vi "state_to_pose.vi"(1 "Handle State":sgl[][](array[numeric])) -> (0 "Pose":T1)   [LabVIEW 2013]
uses:
  <vilib>/Analysis/Matrix/Datatypes/RealMatrix.ctl
  <vilib>/Analysis/Matrix/Numeric/Conversions/Array To Matrix - RA.vi
  <vilib>/Analysis/Matrix/NI_Matrix.lvlib
panel:
  # "Position XYZ (microns)"
  # "Velocity XYZ (mm/sec)"
  # "Acceleration XYZ (m/sec)"
  # "Euler angles (radians)"
  # "Euler rates (radians/sec)"
  # "Given 2D array representation of KF state, convert to pose matrix."
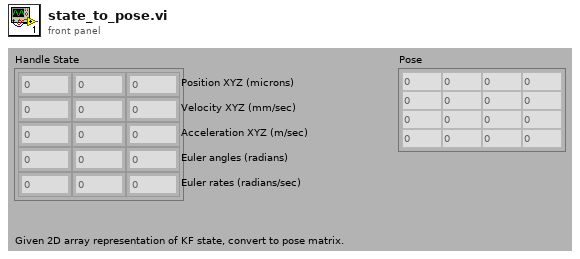
[diagram p1: front panel]
types:
  T1 = typedef "NI_Matrix.lvlib/RealMatrix.ctl" = dbl[][]
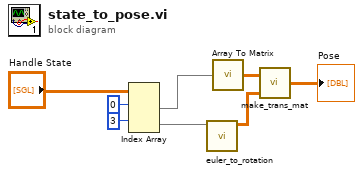
[diagram p0: block diagram]
diagram:
  n1 = Index Array(array="Handle State", index (row) #1=0 ("index (row)"), index (row) #2=3 ("index (row)")) -> (element #1=w7:sgl[], element #2=w8:sgl[])  [unwired: 2 in]
  n2 = call "euler_to_rotation.vi"("Theta XYZ"=w8) -> ("Rotation"=w3:T1)  [unwired: 10 in]
  n3 = call-poly <vilib>:"Array To Matrix.vi"("Real 1D Array"=w7) -> ("Real Matrix (Column Vector)"=w2:T1)
  n4 = call "make_trans_mat.vi"("Rotation"=w3, "Translation"=w2) -> ("Transform"=→"Pose":T1)  [unwired: 3 out]
